vi "初始化编码器位置.vi"(8 "error in (no error)":errorcluster, 11 "原始位置":dbl) -> (0 "error out":errorcluster)   [LabVIEW 2016, in "elevator.lvlib"]
uses:
  elevator.lvlib
  DAM395CF/DAM395CF.lvlib
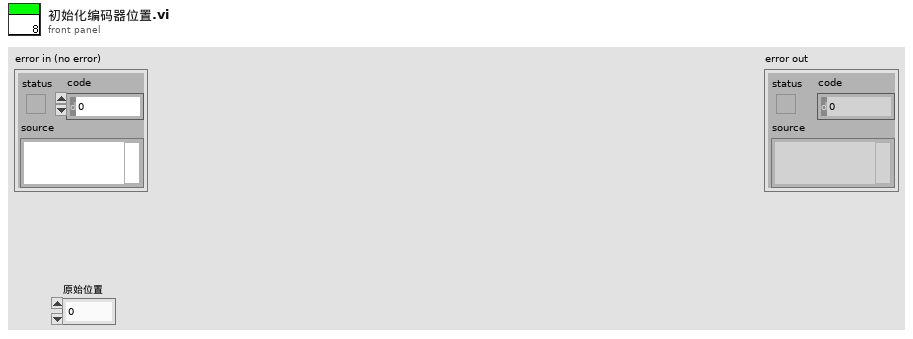
[diagram p1: front panel]
types:
  T1 = enum16{"通道0", "通道1", "通道2", "通道3", "通道4", "通道5", "通道6", "通道7"}
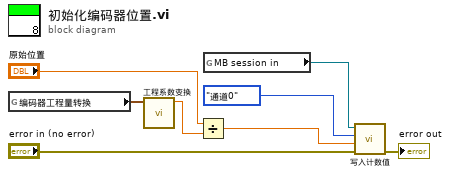
[diagram p0: block diagram]
diagram:
  n1 = global read "elevator 全局变量.vi" "编码器工程量转换"() -> (w4:cluster{"编码器计数值":dbl, "工程计量值":dbl})
  n2 = call "工程系数变换.vi"("编码器工程量转换"=w4) -> ("工程变换系数"=w3:dbl)  [unwired: 10 in]
  n3 = Divide(x="原始位置", y=w3) -> (x/y=w1:dbl)
  n4 = global read "elevator 全局变量.vi" "MB session in"() -> (w8:refnum<class "MB_Master.lvclass">)
  n5 = call "写入计数值.vi"("error in (no error)"="error in (no error)", "计数值"=w1, "通道"=T1."通道0", "MB session in"=w8) -> ("error out"=→"error out":errorcluster)  [unwired: 6 in, 1 out]
